vi "溫度濕度.vi"() -> ()   [LabVIEW 2019]
uses:
  <vilib>/LabVIEW Interface for Arduino/LabVIEW Interface for Arduino.lvlib
panel:
  in  "Analog Input Pin (0)":u8
  in  "stop":bool
  out "Thermometer":dbl(slide) scale=0.0..100.0
  out "Numeric":dbl
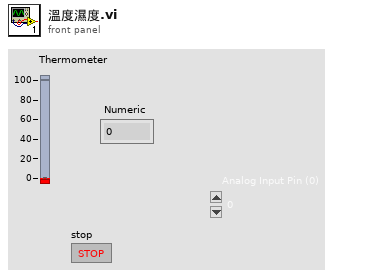
[diagram p1: front panel]
types:
  T1 = typedef "LabVIEW Interface for Arduino.lvlib/Arduino Resource.ctl" = cluster{"VISA resource":refnum<visa-resource-name>, "Board Type":T2, "Connection Type":enum8{"USB / Serial"}, "Bytes Per Packet (15)":u8}
  T2 = typedef "LabVIEW Interface for Arduino.lvlib/Board Type.ctl" = enum16{"Uno", "Dimuelanove w/Atmega 328", "Mega 2560"}
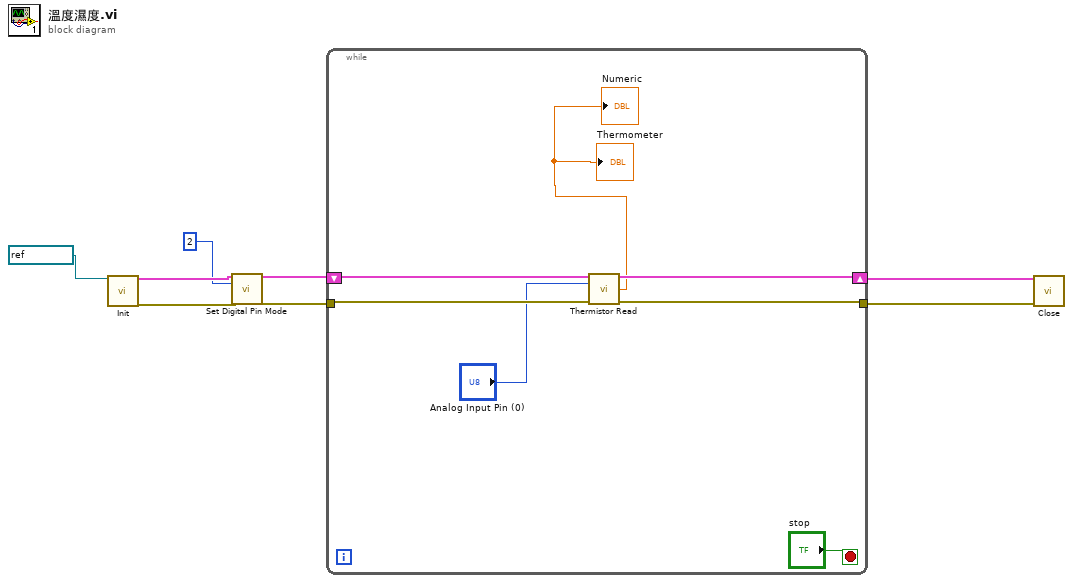
[diagram p0: block diagram]
diagram:
  n1 = call <vilib>:"Init.vi"("VISA resource"=refnum<visa-resource-name> "COM6") -> ("Arduino Resource"=w5:T1, "error out"=w4:errorcluster)  [unwired: 17 in]
  n2 = call <vilib>:"Set Digital Pin Mode.vi"("Arduino Resource"=w5, "Digital I/O Pin"=u8 2, "error in"=w4) -> ("Arduino Resource"=w2:T1, "error out"=w1:errorcluster)  [unwired: 11 in]
  n3 = while {
    tunnel: [w13] -> w6
    shift-right: [w14] -> w7
    shift-left: w2 -> [w11]
    tunnel: w1 -> [w12]
    stop <- "stop" stop-if-true
    n4 = call <vilib>:"Thermistor Read.vi"("Arduino Resource"=w11, "Thermistor AI Pin (0)"="Analog Input Pin (0)", "error in"=w12) -> ("Arduino Resource"=w14:T1, "Temperature"=→"Thermometer" →"Numeric":dbl, "error out"=w13:errorcluster)  [unwired: 10 in]
  }
  n5 = call <vilib>:"Close.vi"("Arduino Resource"=w7, "error in"=w6) -> ()  [unwired: 13 in, 1 out]
